vi "DataBase Search.vi"() -> ()   [LabVIEW 2014]
panel:
  out "transposed array":string[][](array[string])
  out "Match Found":bool
  out "j":i32
  out "Columns":i32
  out "Rows":i32
  in  "Search Item":i8(knob) scale=0.0..2.0
  in  "Search Element":string
  out "i":i32
  # "ELCOM DIAS : DATABASE SEARCH"
  # "Student Details :"
  # "Array Size :"
  # "Name :"
  # "Search Element"
  # "x"
  # "Register Number :"
  # "Name                 :"
  # "Phone Number   :"
  # "Year                    :"
  # "Register\nNumber :"
  # "Phone\nNumber :"
  # "Search Result  :"
  # "Match Found ?"
  # "Element found at ?"
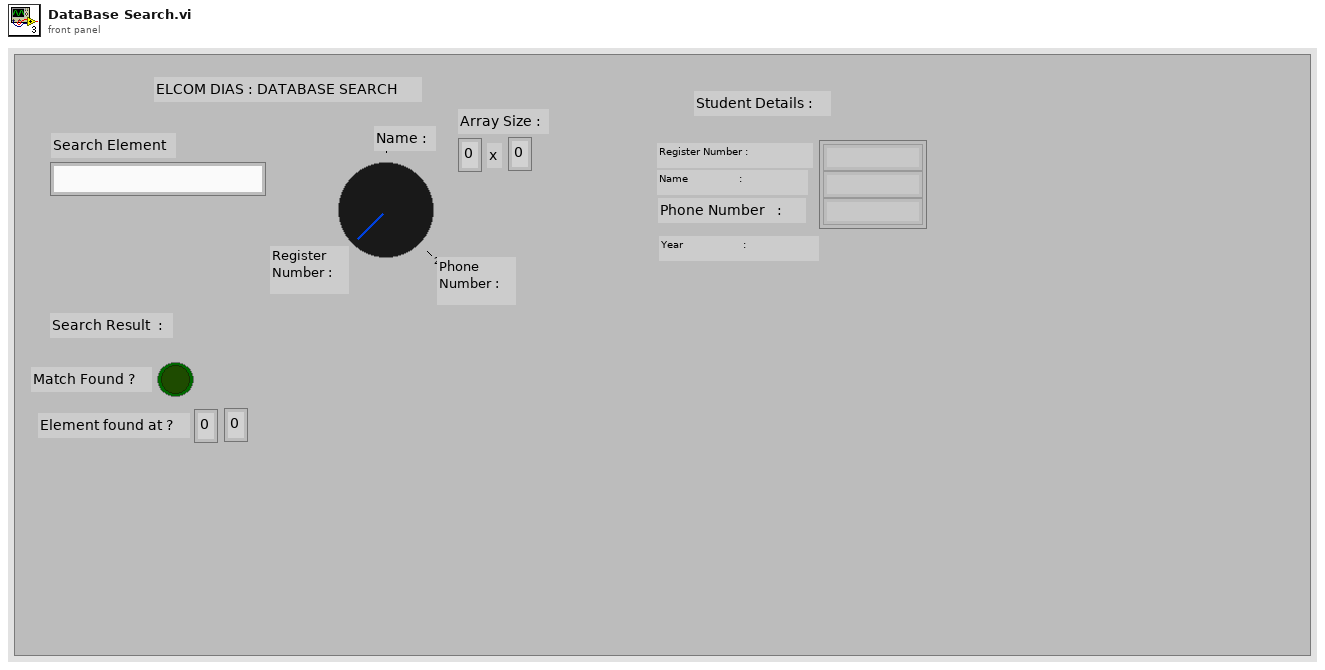
[diagram p1: front panel]
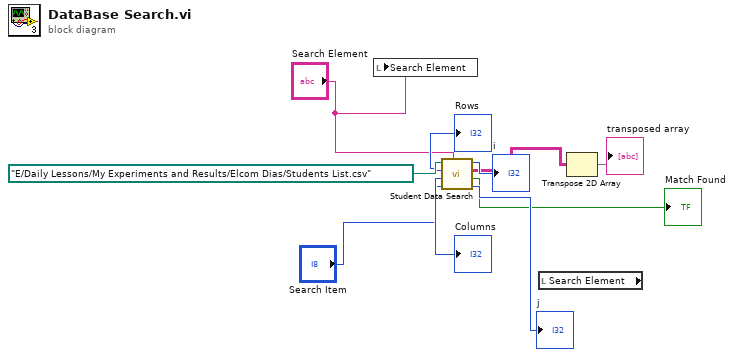
[diagram p0: block diagram]
diagram:
  n1 = local write "Search Element"("Search Element") -> ()
  n2 = call "Student Data Search.vi"("Search Element"="Search Element", "Search Item"="Search Item", "file path (dialog if empty)"=path "E:/Daily Lessons/My Experiments and Results/Elcom Dias/Students List.csv") -> ("j"=→"j":i32, "Match Found"=→"Match Found":bool, "subarray"=w4:string[][], "i"=→"i":i32, "Columns"=→"Columns":i32, "Rows"=→"Rows":i32)
  n3 = local read "Search Element"() -> ()  [unwired: 1 out]
  n4 = Transpose 2D Array(2D array=w4) -> (transposed array=→"transposed array":string[][])
